vi "Cursor Interpolation Example.vi"() -> ()   [LabVIEW 2018]
panel:
  in  "Graph Detail":i32
  in  "Method":i32(ring)=1 items=["nearest", "linear", "spline", "cubic Hermite", "Lagrange"]
  in  "Del Point":bool
  in  "Add Point":bool
  out "XY Graph":cluster{"X":dbl, "Y":dbl}[](graph)
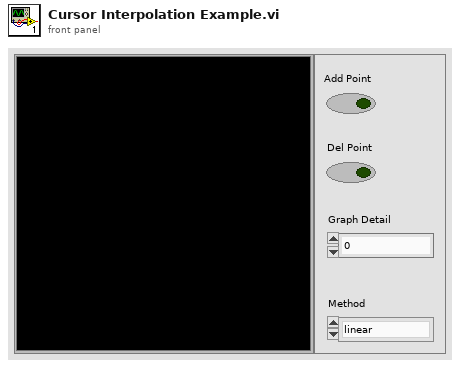
[diagram p1: front panel]
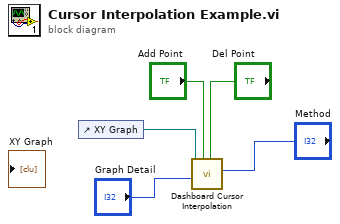
[diagram p0: block diagram]
diagram:
  n1 = control-ref of="XY Graph"() -> (w3:refnum<vi>)
  n2 = call "Dashboard Cursor Interpolation.vi"("Remove Cursor"="Del Point", "Add Cursor"="Add Point", "Graph Detail"="Graph Detail", "Interpolation Method"="Method", "Interpolation Points"=w3) -> ()  [unwired: 7 in]
